vi "002 copia timed loop.vi"() -> ()   [LabVIEW 2019]
uses:
  <vilib>/Platform/TimedLoop/XDataNode/timing_clust.ctl
  <vilib>/Platform/TimedLoop/XDataNode/nitl_modes.ctl
  <vilib>/Platform/TimedLoop/XDataNode/wakeup.ctl
  <vilib>/platform/TimedLoop/XDataNode/XDataNode.xnode
  <vilib>/Platform/TimedLoop/XDataNode/XDNodeRunTimeDep.lvlib
panel:
  out "resta 2":i32
  out "Iteracions 2":i32
  out "Finished Late? [i-1] 2":bool
  out "x > 0? 2":bool
  out "x > 0?":bool
  out "Finished Late? [i-1]":bool
  out "Iteracions":i32
  out "resta":i32
  in  "stop general":bool
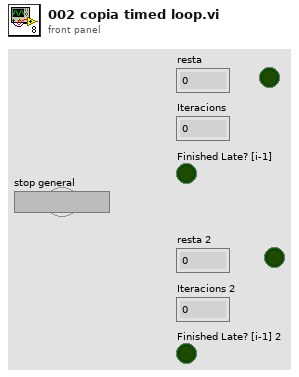
[diagram p1: front panel]
types:
  T1 = typedef "XDNodeRunTimeDep.lvlib/timing_clust.ctl" = cluster{"Expected End [f-1]":u64, "Actual End [f-1]":u64, "Finished Late? [f-1]":bool, "Expected End [i-1]":u64, "Actual End [i-1]":u64, "Finished Late? [i-1]":bool, "Expected Start [i]":u64, "Actual Start [i]":u64, "Expected Start [f]":u64, "Actual Start [f]":u64, "Source Name":string, "Structure Name":string, "Period":i64, "Deadline":i64, "Offset":i64, "Start":i64, "Priority":i32, "Timeout":i32, "Mode":T2, "Wakeup Reason":T3, "Error":errorcluster, "Source Type":string, "Secondary Source Type":string, "Global End Time":u64, "Global Start Time":u64, "Frame Duration":u64, "Iteration Duration":u64, "Assigned CPU":i32, "I/O Scan Engine Mode":u32}
  T2 = typedef "XDNodeRunTimeDep.lvlib/nitl_modes.ctl" = enum32{"No Change", "Process missed periods, maintain original phase", "Discard missed periods, maintain original phase", "Process missed periods, ignore original phase", "Discard missed periods, ignore original phase"}
  T3 = typedef "XDNodeRunTimeDep.lvlib/wakeup.ctl" = enum32{"Normal", "Aborted", "Asynchronous wakeup", "Timing source error", "Timed loop error", "Timeout"}
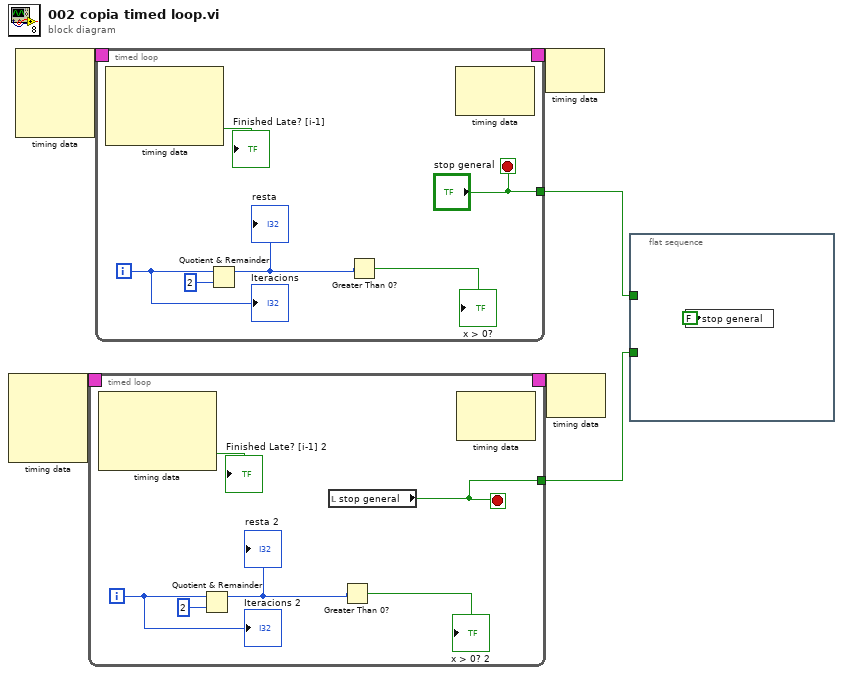
[diagram p0: block diagram]
diagram:
  n1 = node-c288() -> (w4:T1)  [unwired: 4 in]
  n2 = node-c288() -> (w6:T1)  [unwired: 4 in]
  n3 = timed-loop {
    timing: w4 -> [_]
    timing-out: [_] -> w3
    tunnel: [w7] -> w1
    i -> [w12]
    stop <- w7 stop-if-true
    n4 = node-c288() -> (→"Finished Late? [i-1] 2":bool)  [unwired: 1 in, 3 out]
    n5 = Quotient & Remainder(x=w12, y=2) -> (x-y*floor(x/y)=w9:i32)  [unwired: 1 out]
    "resta 2" <- w9
    n6 = local read "stop general"() -> (w7:bool)
    n7 = Greater Than 0?(x=w9) -> (x > 0?=→"x > 0? 2":bool)
    n8 = node-c288() -> ()  [unwired: 2 in, 1 out]
    "Iteracions 2" <- w12
  }
  n9 = timed-loop {
    timing: w6 -> [_]
    timing-out: [_] -> w5
    tunnel: ["stop general"] -> w2
    i -> [w21]
    stop <- "stop general" stop-if-true
    n10 = node-c288() -> (→"Finished Late? [i-1]":bool)  [unwired: 1 in, 3 out]
    n11 = Quotient & Remainder(x=w21, y=2) -> (x-y*floor(x/y)=w18:i32)  [unwired: 1 out]
    "resta" <- w18
    n12 = Greater Than 0?(x=w18) -> (x > 0?=→"x > 0?":bool)
    n13 = node-c288() -> ()  [unwired: 2 in, 1 out]
    "Iteracions" <- w21
  }
  n14 = node-c288(w5) -> ()  [unwired: 1 out]
  n15 = node-c288(w3) -> ()  [unwired: 1 out]
  n16 = flat-sequence {
    tunnel: w2 -> [_]
    tunnel: w1 -> [_]
    frame #0 {
      n17 = local write "stop general"(FALSE ("stop")) -> ()
    }
  }
